vi "SCCSup Dialog_GenMCLB_PadColumn.vi"(8 "error in (no error)":errorcluster, 9 "padding":u32, 10 "column":i32, 11 "multicolumn listbox":refnum<vi>) -> (0 "error out":errorcluster)   [LabVIEW 2017]
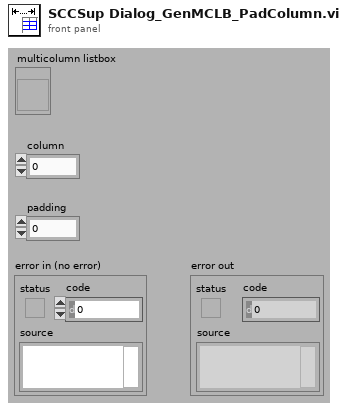
[diagram p1: front panel]
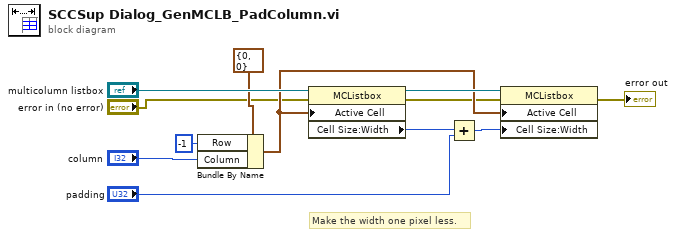
[diagram p0: block diagram]
diagram:
  # "Make the width one pixel less."
  n1 = Bundle By Name(cluster=cluster{"Row":i32, "Column":i32} {"Row"=0, "Column"=0} ("Active Cell"), "Row"=-1, "Column"="column") -> (w9:cluster{"Row":i32, "Column":i32})
  n2 = property on="Property Node" class="MCListbox"(reference="multicolumn listbox", error in="error in (no error)", "Active Cell"=w9) -> (reference out=w10:refnum<vi>, error out=w4:errorcluster, "Cell Size:Width"=w8:u32)
  n3 = Add(x=w8, y="padding") -> (x+y=w7:u32)
  n4 = property on="Property Node" class="MCListbox"(reference=w10, error in=w4, "Active Cell"=w9, "Cell Size:Width"=w7) -> (error out=→"error out":errorcluster)  [unwired: 1 out]
